vi "test_main.vi"() -> ()   [LabVIEW 2016]
uses:
  AutoBike/Typedef/Remote Control Cluster.ctl
  Downloads/PID Gains.ctl
  LabView Navigation/INS Data.ctl
  <vilib>/FPGAPlugInAG/roboRIO/niLvFpga_Open_roboRIO.vi
  <vilib>/rvi/interface/common/dynamic/niFpgaDynamicAddResources.vi
  <vilib>/FPGAPlugInAG/Dynamic/niLvFpga_Reset_Dynamic.vi
  <vilib>/Utility/error.llb/Error Cluster From Error Code.vi
  <vilib>/rvi/errors/niLvFpgaAdjustHostInterfaceError.vi
  <vilib>/myRIO/Common/Instrument Driver Framework/Utilities/vis/FPGA Ref Manager.vi
  <vilib>/myRIO/Common/Instrument Driver Framework/Utilities/vis/Ref Counter.vi
  <vilib>/FPGAPlugInAG/Dynamic/niLvFpga_Run_Dynamic.vi
  <vilib>/RVI Host/nirviSupport.llb/nirviErrorClusterFromErrorCode.vi
  <vilib>/addons/control/pid/pid.llb/PID (DBL).vi
  <vilib>/Utility/file.llb/Read Delimited Spreadsheet (DBL).vi
  <vilib>/rvi/interface/nirviOpenFPGA/nirviOpenFPGA.xnode
  AutoBike/FPGA Bitfiles/AutoBikeMainFPGAbitfile.lvbitx
  <vilib>/rvi/interface/nirviMethod/nirviMethod.xnode
  <vilib>/rvi/interface/nirviReadWriteControl/nirviReadWriteControl.xnode
  <vilib>/ErrorRing/Error Ring.xnode
  <vilib>/rvi/interface/Simulation/niFpgaSimulationCallBeginRW.vi
  NiFpgaLv.dll
  <vilib>/FPGAPlugInAG/Dynamic/niLvFpga_WriteFifo_Dynamic.vi
  <vilib>/rvi/errors/niLvFpgaMergeErrorWithErrorCode.vi
  <vilib>/rvi/interface/nirviMethod/StockFPGA_InlinedMethodWaitForSingleIRQ.vi
  <vilib>/FPGAPlugInAG/Dynamic/niLvFpga_WaitOnIrq_Dynamic.vi
  <vilib>/FPGAPlugInAG/Dynamic/niLvFpga_AcknowledgeIrq_Dynamic.vi
  <vilib>/addons/control/pid/NI_PID_pid.lvlib
  <vilib>/myRIO/Instrument Drivers/Utilities/Utilities.lvlib
  <vilib>/FPGAPlugInAG/Dynamic/niLvFpga_StartFifo_Dynamic.vi
  <vilib>/FPGAPlugInAG/Dynamic/niLvFpga_ReadFifo_Dynamic.vi
panel:
  out "Increment Lean":i8
  out "PositionData":T1
  out "SteeringAngle(deg)":dbl
  out "all rows":dbl[][](array[numeric])
  out "Delta Heading":dbl
  in  "useUWB":bool=TRUE
  out "X_UWB":dbl
  out "Y_UWB":dbl
  out "Z_UWB":dbl
  in  "Send vel":bool
  out "VEL":u16=850
  in  "resetPID":bool
  in  "PID gains":T2={"proportional gain (Kc)"=-3.418, "integral time (Ti, min)"=45.215, "derivative time (Td, min)"=0.0011} {"derivative time (Td, min)" format="%.8f"; "integral time (Ti, min)" format="%.8f"; "proportional gain (Kc)" format="%.8f"}
  in  "Gear":enum16{"7", "6", "5", "4", "3", "2", "1"}(ring)=enum."4"
  in  "maxDiff":dbl=0.75
  out "km/h":sgl
  out "Setpoint":dbl
  out "Set Roll":dbl(graph)
  out "encoder setpoint":i16(graph)
  out "Roll":sgl(graph)
  in  "Reset Errors":bool
  out "ODrive State":u8
  out "ODrive Errors":u32
  out "ODrive Error Flags":bool[](array[boolean])
  out "Position Axis1":i16
  out "Velocity Axis0":i16
  out "Remote Control Data":T3
  out "Encoder Index Position":i16
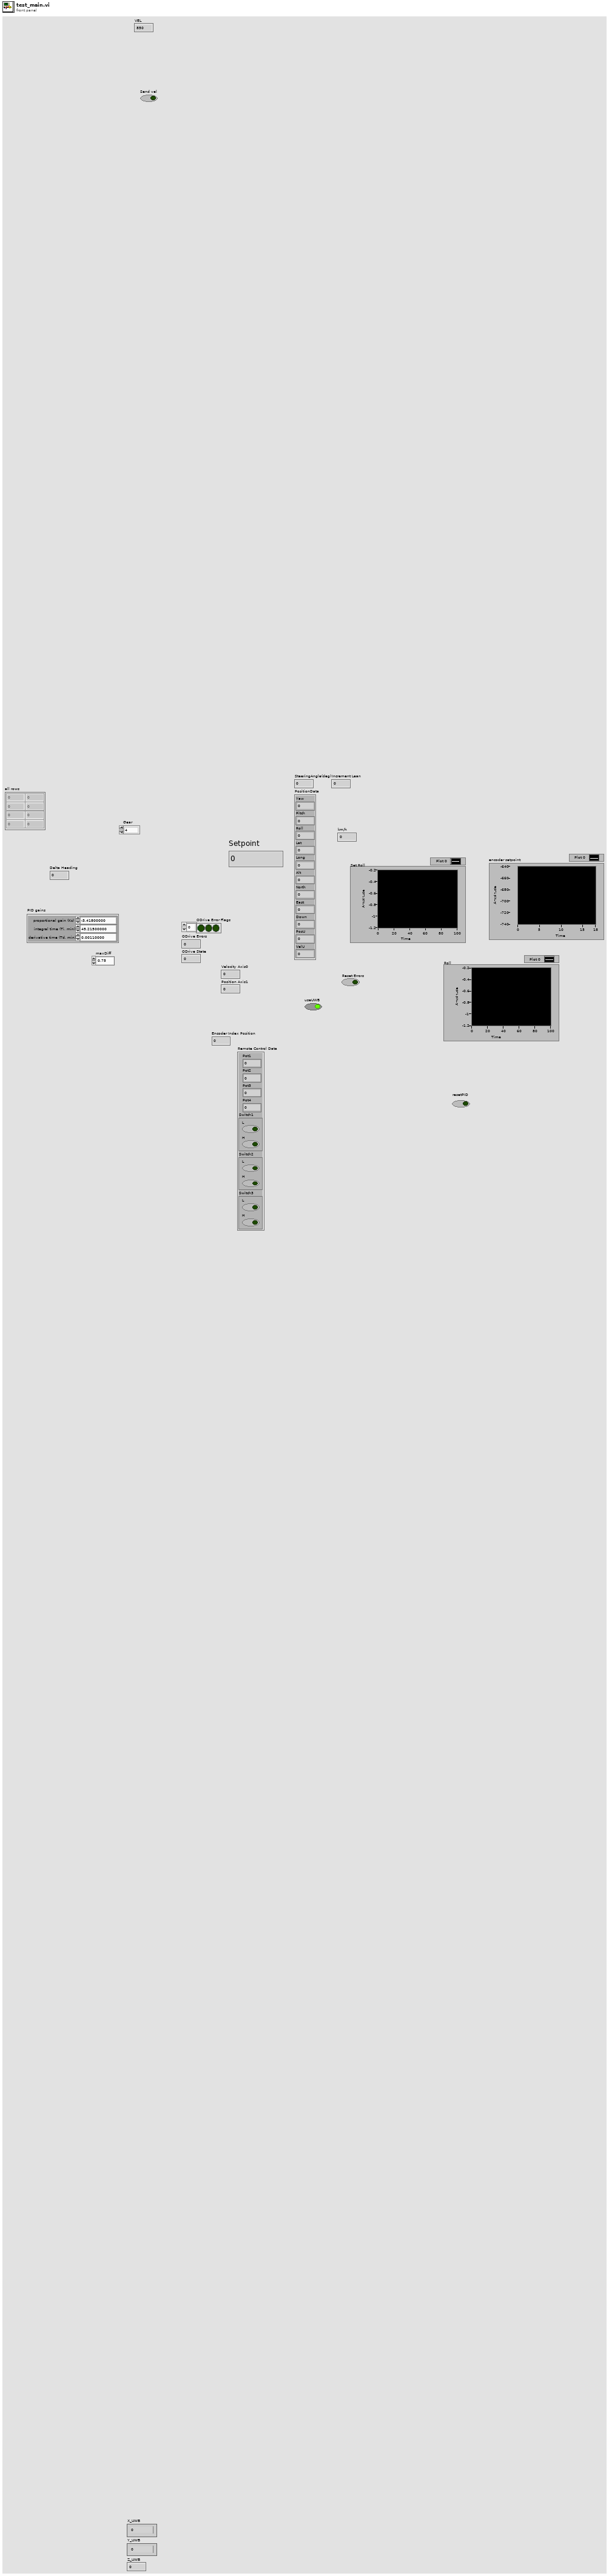
[diagram p1: front panel]
types:
  T1 = typedef "INS Data.ctl" = cluster{"Yaw":sgl, "Pitch":sgl, "Roll":sgl, "Lat":dbl, "Long":dbl, "Alt":dbl, "North":dbl, "East":dbl, "Down":dbl, "PosU":dbl, "VelU":dbl}
  T2 = typedef "PID Gains.ctl" = cluster{"proportional gain (Kc)":dbl, "integral time (Ti, min)":dbl, "derivative time (Td, min)":dbl}
  T3 = typedef "Remote Control Cluster.ctl" = cluster{"Pot1":u16, "Pot2":u16, "Pot3":u16, "Pot4":u16, "Switch1":cluster{"L":bool, "H":bool}, "Switch2":cluster{"L":bool, "H":bool}, "Switch3":cluster{"L":bool, "H":bool}}
  T4 = typedef "Semaphore RefNum" = refnum<k1>
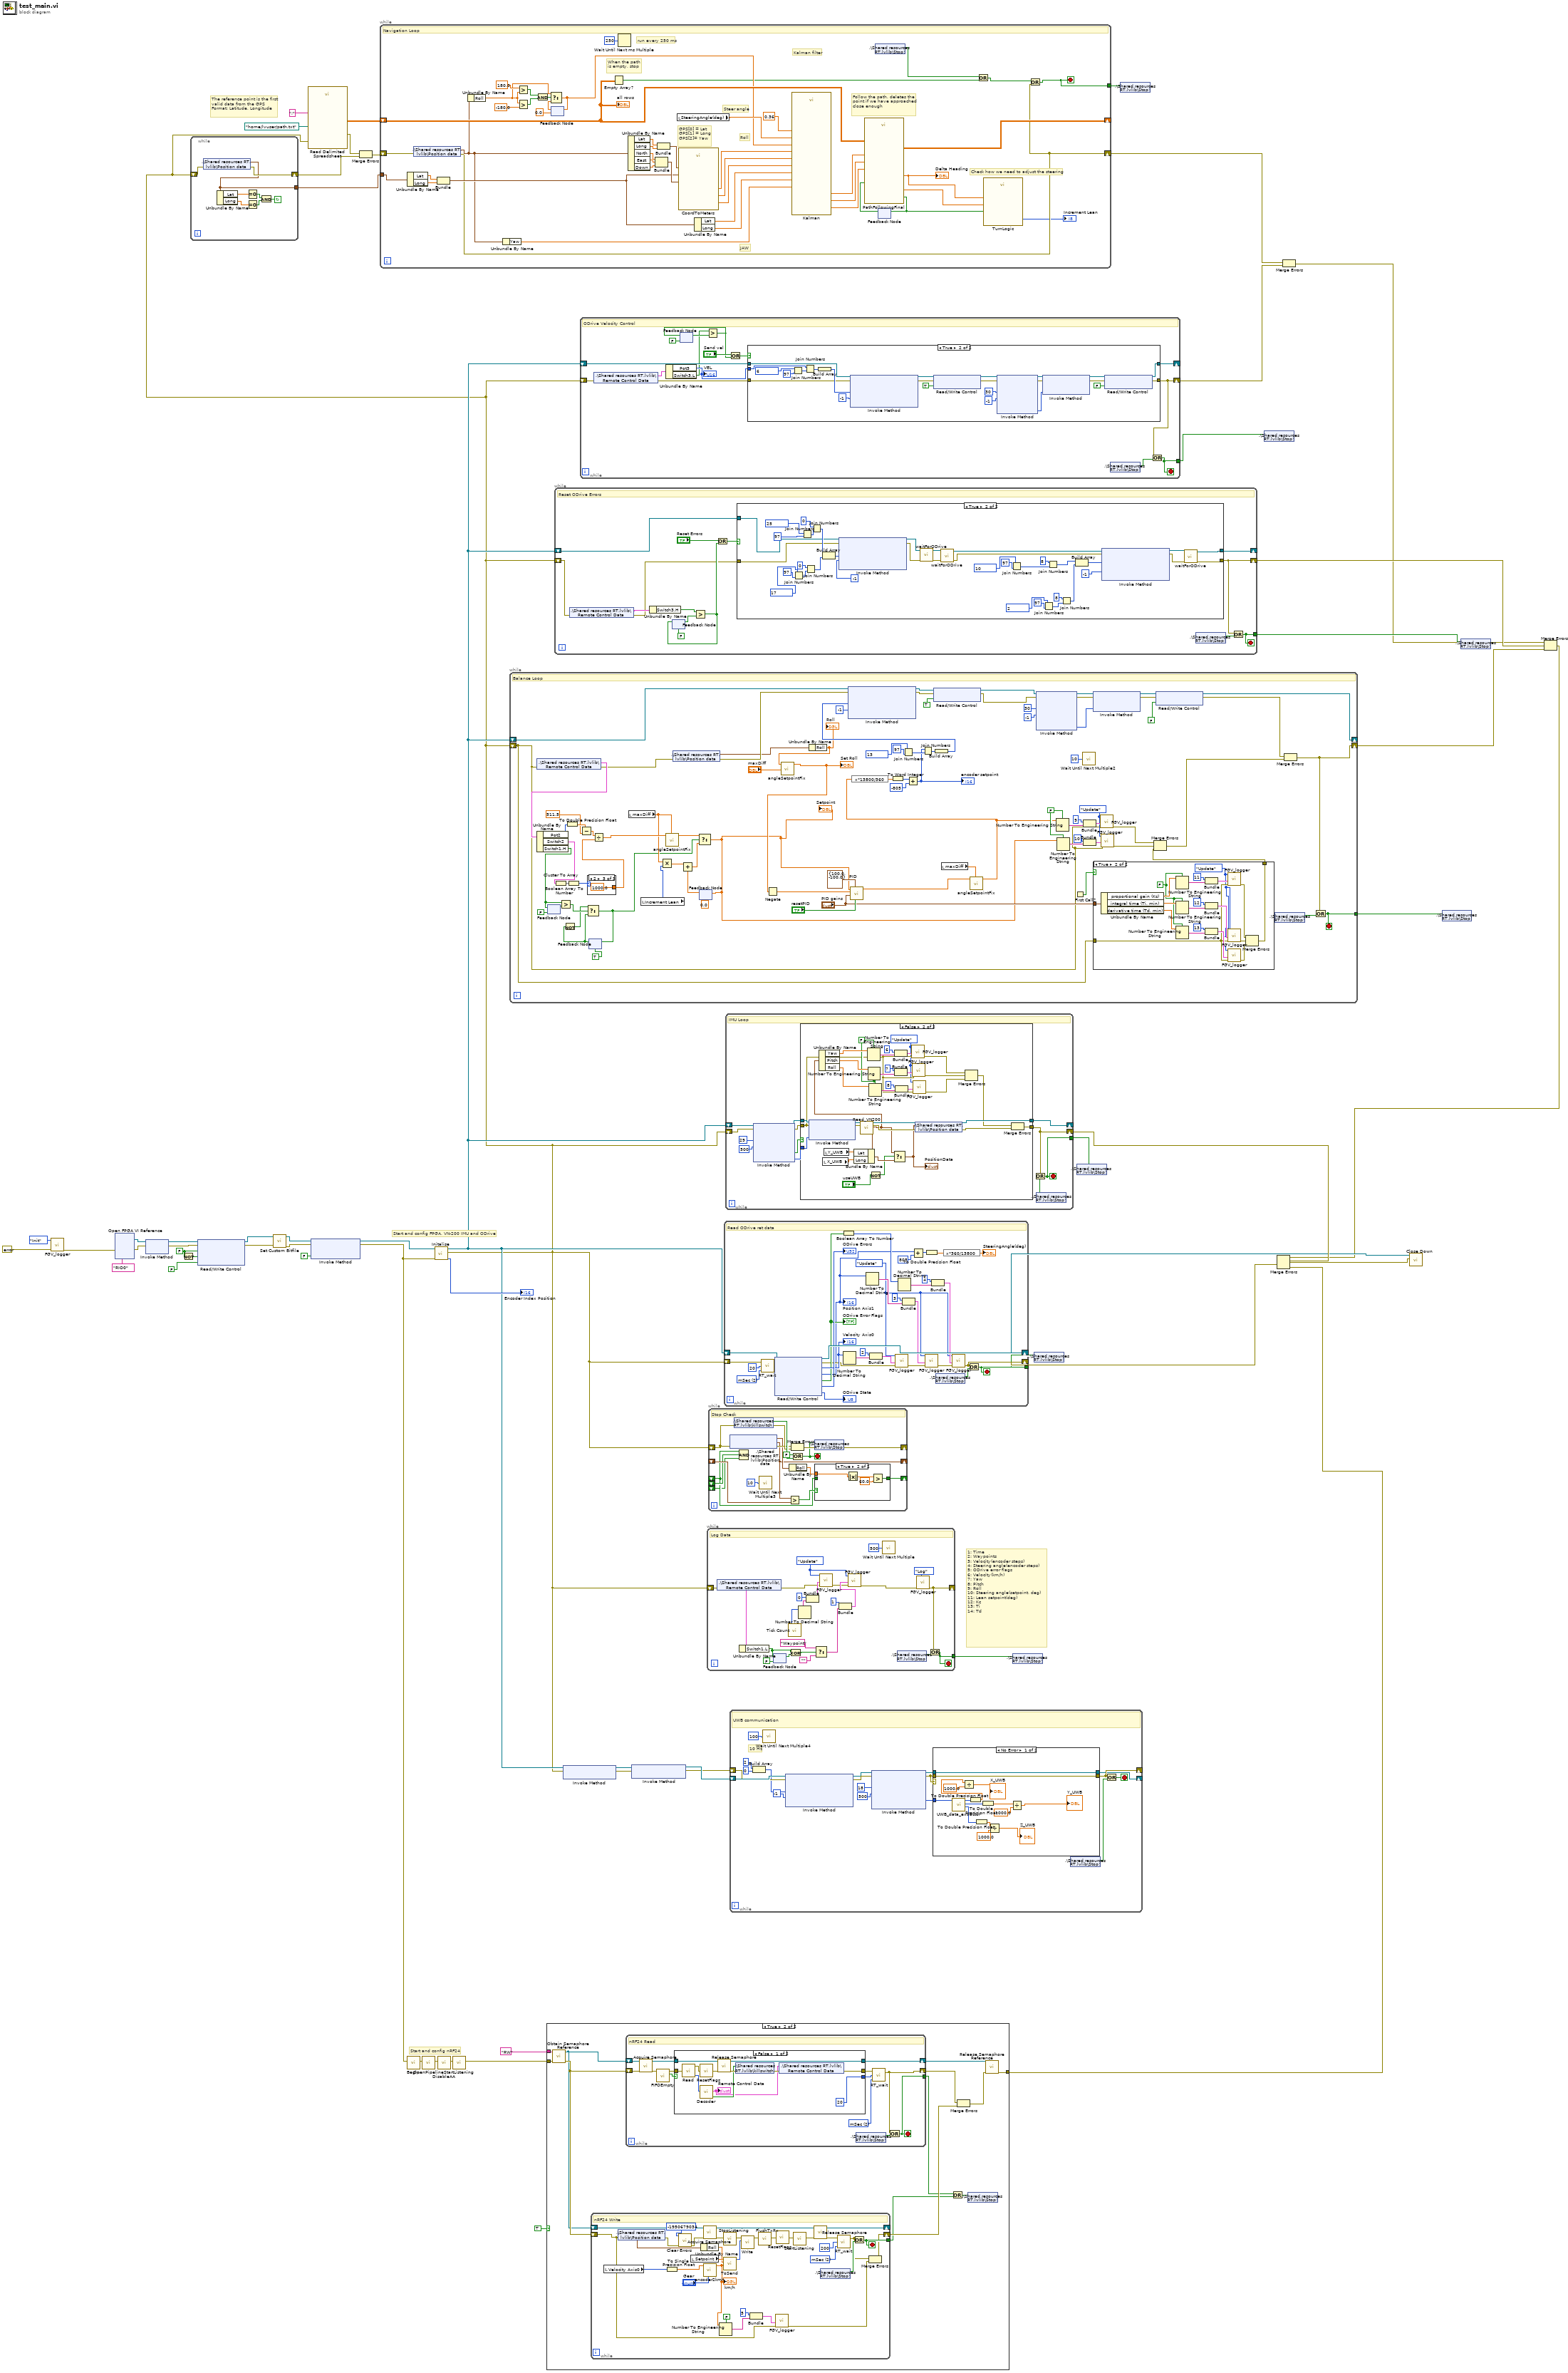
[diagram p0: block diagram]
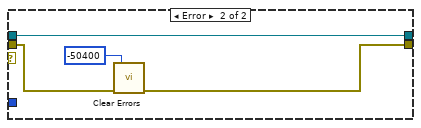
[diagram p2: hidden frame]
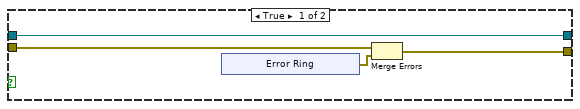
[diagram p3: hidden frame]
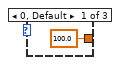
[diagram p8: hidden frame]
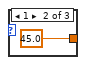
[diagram p9: hidden frame]
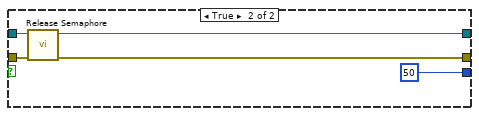
[diagram p11: hidden frame]
diagram:
  w29 = FALSE ("Steering motor on?")
  # "The reference point is the first valid data from the GPS\nFormat: Latitude, Longitude"
  # "1: Time\n2: Waypoints\n3: Velocity(encoder steps)\n4: Steering angle(encoder steps)\n5: ODrive error flags\n6: Velocity(km/h)\n7: Yaw\n8: Pitch\n9: Roll\n10: Steering angle(setpoint, deg)\n11: Lean setpoint(deg)\n12: Kc\n13: Ti\n14: Td"
  # "Start and config FPGA, VN-200 IMU and ODrive"
  # "Start and config nRF24"
  n1 = call "FGV_logger.vi"("error in"=errorcluster {"status"=FALSE, "code"=0, "source"=""}, "Command"=enum16{"Update", "Log", "Init"}."Init") -> ("error out"=w36:errorcluster)  [unwired: 9 in]
  n2 = xnode "Open FPGA VI Reference"("error in"=w36, "resource name"=tag "RIO0") -> ("FPGA VI Reference Out"=w20:refnum<k20>, "error out"=w21:errorcluster)
  n3 = xnode "Invoke Method"("FPGA VI Reference In"=w20, "error in"=w21) -> ("FPGA VI Reference Out"=w33:refnum<k20>, "error out"=w32:errorcluster)
  n4 = Not(x=w29) -> (.not. x?=w30:bool)
  n5 = xnode "Read/Write Control"("FPGA VI Reference In"=w33, "error in"=w32, "Comm LED Green"=w29, "Comm LED Red"=w30, "MotorsON"=FALSE ("Rear wheel motor OFF?")) -> ("FPGA VI Reference Out"=w26:refnum<k20>, "error out"=w27:errorcluster)
  n6 = call <vilib>:"Set Custom Bitfile.vi"("error in (no error)"=w27, "Custom FPGA Reference In"=w26) -> ("error out"=w25:errorcluster, "Custom FPGA Reference Out"=w24:refnum<k20>)  [unwired: 8 in]
  n7 = xnode "Invoke Method"("FPGA VI Reference In"=w24, "error in"=w25, "Wait Until Done (F)"=FALSE) -> ("FPGA VI Reference Out"=w22:refnum<k20>, "error out"=w23:errorcluster)
  n8 = call "Begin.vi"("error in (no error)"=w23) -> ("error out"=w41:errorcluster)  [unwired: 10 in]
  n9 = call "OpenPipeline.vi"("error in (no error)"=w41) -> ("error out"=w40:errorcluster)  [unwired: 10 in]
  n10 = call "Initalise.vi"("error in (no error)"=w23, "FPGA Interface"=w22) -> ("Encoder Index Position"=→"Encoder Index Position":i16, "Error out"=w7:errorcluster, "FPGA VI Reference Out"=w13:refnum<k20>)  [unwired: 7 in]
  n11 = while {
    shift-right: [w64] -> w8
    shift-left: w7 -> [w63]
    tunnel: [w57] -> w9
    stop <- w58 continue-if-true
    n12 = shared-variable ".\\Shared resources RT.lvlib\\Position data"(error in=w63) -> (w57:T1, error out=w64:errorcluster)
    n13 = Unbundle By Name(w57) -> ("Lat"=w62:dbl, "Long"=w61:dbl)
    n14 = Equal To 0?(x=w62) -> (x = 0?=w60:bool)
    n15 = Equal To 0?(x=w61) -> (x = 0?=w59:bool)
    n16 = And(x=w60, y=w59) -> (x .and. y?=w58:bool)
  }
  n17 = call-poly <vilib>:"Read Delimited Spreadsheet.vi"("file path (dialog if empty)"=path "/home/lvuser/path.txt", "error in (no error)"=w7, "delimiter (\\t)"=";" ("delimiter (\\t)")) -> ("all rows"=w10:dbl[][], "error out"=w6:errorcluster)  [unwired: 7 in, 4 out]
  n18 = Merge Errors(w6, w8) -> (w5:errorcluster)
  n19 = while {
    shift-right: [w109] -> _
    shift-left: w10 -> [w97]
    tunnel: w9 -> [w76]
    shift-right: [w70] -> w1
    shift-left: w5 -> [w71]
    tunnel: [w66] -> w4
    stop <- w66 stop-if-true
    # "Roll"
    # "Steer angle"
    # "JAW"
    # "Check how we need to adjust the steering"
    # "Kalman filter"
    # "run every 250 ms"
    # "Follow the path, deletes the point if we have approached close enough"
    # "GPS[0] = Lat\nGPS[1] = Long \nGPS[2]= Yaw"
    # "When the path is empty, stop"
    # "Navigation Loop"
    n20 = Unbundle By Name(w76) -> ("Lat"=w75:dbl, "Long"=w74:dbl)
    n21 = shared-variable ".\\Shared resources RT.lvlib\\Position data"(error in=w71) -> (w72:T1, error out=w70:errorcluster)
    n22 = Bundle("Lat"=w75, "Long"=w74) -> (w73:cluster{"Lat":dbl, "Long":dbl})  [unwired: 1 in]
    n23 = Unbundle By Name(w72) -> ("Roll"=w81:sgl)
    n24 = Unbundle By Name(w72) -> ("Yaw"=w77:sgl)
    n25 = Greater?(x=sgl 180.0 ("upper limit"), y=w81) -> (0:w82:bool)
    n26 = Greater?(x=w81, y=sgl -180.0 ("lower limit")) -> (0:w84:bool)
    n27 = And(x=w82, y=w84) -> (x .and. y?=w83:bool)
    n28 = feedback #1(sgl 0.0 ("Roll")) -> (w80:sgl)
    n29 = Select(t=w81, s=w83, f=w80) -> (s? t:f=w78:sgl)
    n30 = feedback-in #1(w78) -> ()
    n31 = Empty Array?(array=w97) -> (empty?=w69:bool)
    n32 = Wait Until Next ms Multiple(millisecond multiple=u32 250) -> ()  [unwired: 1 out]
    n33 = Unbundle By Name(w72) -> ("Lat"=w104:dbl, "Long"=w103:dbl, "North"=w101:dbl, "East"=w100:dbl, "Down"=w99:dbl)
    n34 = Bundle("North"=w101, "East"=w100, "Down"=w99) -> (w98:cluster{"North":dbl, "East":dbl, "Down":dbl})  [unwired: 1 in]
    n35 = Bundle("Lat"=w104, "Long"=w103) -> (w102:cluster{"Lat":dbl, "Long":dbl})  [unwired: 1 in]
    n36 = local read "SteeringAngle(deg)"() -> (w87:dbl)
    n37 = call "CoordToMeters.vi"("VelNed"=w98, "Ref Point"=w73, "GPS position"=w102) -> ("Bike Heading"=w94:dbl, "X"=w95:dbl, "Y"=w96:dbl)  [unwired: 6 in]
    n38 = Unbundle By Name(w73) -> ("Lat"=w89:dbl, "Long"=w88:dbl)
    n39 = call "Kalman.vi"("x"=w88, "y"=w89, "theta"=w77, "GPS X"=w95, "GPS Y"=w96, "GPS theta"=w94, "ds"=0.36, "phi"=w78, "delta"=w87) -> ("new x"=w91:dbl, "new y"=w92:dbl, "new theta"=w90:dbl)  [unwired: 8 in]
    n40 = shared-variable ".\\Shared resources RT.lvlib\\Stop!"() -> (w67:bool)  [unwired: 1 in, 1 out]
    n41 = feedback #2() -> (w108:bool)  [unwired: 1 in]
    n42 = call "PathFollowingFinal.vi"("GPS_Lat"=w92, "GPS_Long"=w91, "Path"=w97, "Heading angle"=w90, "Save heading"=w108) -> ("Path rest"=w109:dbl[][], "Delta Heading Angle"=w106:dbl, "Goal reached"=w105:bool, "Beta"=w107:dbl)  [unwired: 7 in]
    "Delta Heading" <- w106
    n43 = feedback-in #2(w105) -> ()
    n44 = Or(x=w67, y=w69) -> (x .or. y?=w68:bool)
    n45 = call "TurnLogic.vi"("Goal Reached"=w105, "Beta"=w107, "Delta Theta"=w106) -> ("Increment Lean"=→"Increment Lean":i8)  [unwired: 8 in]
    n46 = Or(x=w68, y=w70) -> (x .or. y?=w66:bool)
    "all rows" <- w97
  }
  n47 = call "DisableAA.vi"("error in (no error)"=w40) -> ("error out"=w39:errorcluster)  [unwired: 10 in]
  n48 = call "StartListening.vi"("error in (no error)"=w39) -> ("error out"=w38:errorcluster)  [unwired: 10 in]
  n49 = while {
    shift-right: [w192] -> _
    shift-left: w13 -> [w193]
    shift-right: [w132] -> w43
    shift-left: w7 -> [w129]
    tunnel: [w154] -> w46
    stop <- w154 stop-if-true
    w138 = enum16{"Update", "Log", "Init"}."Update" ("Command")
    w139 = FALSE ("use system decimal point (T)")
    # "Balance Loop"
    n50 = shared-variable ".\\Shared resources RT.lvlib\\Remote Control Data"(error in=w129) -> (w153:T3, error out=w148:errorcluster)
    n51 = Unbundle By Name(w153) -> ("Pot2"=w189:u16, "Switch2"=w152:cluster{"L":bool, "H":bool}, "Switch1.H"=w118:bool)
    n52 = feedback-in #3(w118) -> ()
    n53 = feedback #3(FALSE ("H")) -> (w117:bool)
    n54 = Cluster To Array(cluster=w152) -> (array=w151:bool[])
    n55 = Greater?(x=w118, y=w117) -> (0:w115:bool)
    n56 = To Double Precision Float(number=w189) -> (double precision float=w187:dbl)
    n57 = Boolean Array To Number(Boolean array=w151) -> (number=w150:u32)
    n58 = Subtract(x=w187, y=511.5 ("x")) -> (x-y=w188:dbl)
    n59 = case shown="2" w150 {
      tunnel: [100.0 45.0 1000.0] -> w149
      frame 0, Default {
      }
      frame 1 {
      }
      frame 2 {
      }
    }
    n60 = feedback #4(TRUE) -> (w113:bool)
    n61 = Not(x=w113) -> (.not. x?=w112:bool)
    n62 = Select(t=w112, s=w115, f=w113) -> (s? t:f=w111:bool)
    n63 = feedback-in #4(w111) -> ()
    n64 = Divide(x=w188, y=w149) -> (x/y=w190:dbl)
    n65 = local read "maxDiff"() -> (w123:dbl)
    n66 = local read "Increment Lean"() -> (w122:i8)
    n67 = Multiply(x=w123, y=w122) -> (x*y=w121:dbl)
    n68 = call "angleSetpointFix.vi"("maxDiff"=w123, "Angle in"=w190) -> ("Angle out"=w126:dbl)  [unwired: 9 in]
    n69 = shared-variable ".\\Shared resources RT.lvlib\\Position data"(error in=w148) -> (w146:T1, error out=w147:errorcluster)
    n70 = feedback #5(0.0 ("Angle out")) -> (w124:dbl)
    n71 = Add(x=w121, y=w124) -> (x+y=w120:dbl)
    n72 = Select(t=w126, s=w111, f=w120) -> (s? t:f=w125:dbl)
    "Setpoint" <- w125
    n73 = feedback-in #5(w125) -> ()
    n74 = Unbundle By Name(w146) -> ("Roll"=w161:sgl)
    "Roll" <- w161
    n75 = call "angleSetpointFix.vi"("maxDiff"="maxDiff", "Angle in"=w161) -> ("Angle out"=w162:dbl)  [unwired: 9 in]
    "Set Roll" <- w162
    n76 = Negate(x=w162) -> (-x=w157:dbl)
    n77 = call-poly <vilib>:"PID.vi"("reinitialize? (F)"="resetPID", "output range"=cluster{"output high":dbl, "output low":dbl} {"output high"=100.0, "output low"=-100.0}, "PID gains"="PID gains", "process variable"=w157, "setpoint"=w125) -> ("output"=w156:dbl)  [unwired: 5 in, 1 out]
    n78 = Join Numbers(hi=u8 13 ("lo"), lo=u8 97) -> ((hi.lo)=w170:u16)
    n79 = local read "maxDiff"() -> (w163:dbl)
    n80 = call "angleSetpointFix.vi"("maxDiff"=w163, "Angle in"=w156) -> ("Angle out"=w135:dbl)  [unwired: 9 in]
    n81 = expression code="x*13800/360"(w135) -> (w164:dbl)
    n82 = To Word Integer(number=w164) -> (16bit integer=w167:i16)
    n83 = Add(x=w167, y=i16 -805 ("hi")) -> (x+y=w165:i16)
    "encoder setpoint" <- w165
    n84 = Join Numbers(hi=w165, lo=w170) -> ((hi.lo)=w169:u32)
    n85 = Build Array(w169) -> (w166:u32[])
    n86 = xnode "Invoke Method"("FPGA VI Reference In"=w193, "error in"=w147, "Data"=w166, "Timeout (ms)"=-1) -> ("FPGA VI Reference Out"=w178:refnum<k20>, "error out"=w179:errorcluster)  [unwired: 1 out]
    n87 = xnode "Read/Write Control"("FPGA VI Reference In"=w178, "error in"=w179, "ODrive RT Control"=TRUE) -> ("FPGA VI Reference Out"=w177:refnum<k20>, "error out"=w176:errorcluster)
    n88 = xnode "Invoke Method"("FPGA VI Reference In"=w177, "error in"=w176, "IRQ Number(s)"=30, "Timeout (ms)"=-1) -> ("FPGA VI Reference Out"=w185:refnum<k20>, "error out"=w184:errorcluster, "IRQ(s) Asserted"=w174:i32)  [unwired: 1 out]
    n89 = Number To Engineering String(1:w139, 4:w135) -> (0:w143:string)  [unwired: 2 in]
    n90 = Number To Engineering String(1:w139, 4:w125) -> (0:w140:string)  [unwired: 2 in]
    n91 = First Call?() -> (First Call?: T/F=w131:bool)
    n92 = call "Wait Until Next Multiple2"("Count(mSec)"=u32 10) -> ()  [unwired: 1 out]
    n93 = Bundle(9, w143) -> (w144:cluster{i32, string})  [unwired: 1 in]
    n94 = Bundle(10, w140) -> (w141:cluster{i32, string})  [unwired: 1 in]
    n95 = case shown="True" w131 {
      tunnel: "PID gains" -> [_ w211]
      tunnel: w129 -> [w194 w200]
      tunnel: [w194 w196] -> w128
      frame False {
      }
      frame True {
        w195 = enum16{"Update", "Log", "Init"}."Update" ("Command")
        w201 = FALSE ("use system decimal point (T)")
        n96 = Unbundle By Name(w211) -> ("proportional gain (Kc)"=w210:dbl, "integral time (Ti, min)"=w203:dbl, "derivative time (Td, min)"=w202:dbl)
        n97 = Number To Engineering String(1:w201, 4:w210) -> (0:w212:string)  [unwired: 2 in]
        n98 = Number To Engineering String(1:w201, 4:w203) -> (0:w207:string)  [unwired: 2 in]
        n99 = Number To Engineering String(1:w201, 4:w202) -> (0:w204:string)  [unwired: 2 in]
        n100 = Bundle(11, w212) -> (w213:cluster{i32, string})  [unwired: 1 in]
        n101 = Bundle(12, w207) -> (w208:cluster{i32, string})  [unwired: 1 in]
        n102 = Bundle(13, w204) -> (w205:cluster{i32, string})  [unwired: 1 in]
        n103 = call "FGV_logger.vi"("error in"=w200, 9:w213, "Command"=w195) -> ("error out"=w199:errorcluster)  [unwired: 8 in]
        n104 = call "FGV_logger.vi"("error in"=w200, 9:w208, "Command"=w195) -> ("error out"=w198:errorcluster)  [unwired: 8 in]
        n105 = call "FGV_logger.vi"("error in"=w200, 9:w205, "Command"=w195) -> ("error out"=w197:errorcluster)  [unwired: 8 in]
        n106 = Merge Errors(w199, w198, w197) -> (w196:errorcluster)
      }
    }
    n107 = xnode "Invoke Method"("FPGA VI Reference In"=w185, "error in"=w184, "IRQ Number(s)"=w174) -> ("FPGA VI Reference Out"=w182:refnum<k20>, "error out"=w173:errorcluster)
    n108 = call "FGV_logger.vi"("error in"=w129, 9:w144, "Command"=w138) -> ("error out"=w137:errorcluster)  [unwired: 8 in]
    n109 = call "FGV_logger.vi"("error in"=w129, 9:w141, "Command"=w138) -> ("error out"=w136:errorcluster)  [unwired: 8 in]
    n110 = Merge Errors(w137, w136, w128) -> (w133:errorcluster)
    n111 = xnode "Read/Write Control"("FPGA VI Reference In"=w182, "error in"=w173, "ODrive RT Control"=FALSE) -> ("FPGA VI Reference Out"=w192:refnum<k20>, "error out"=w134:errorcluster)
    n112 = shared-variable ".\\Shared resources RT.lvlib\\Stop!"() -> (w155:bool)  [unwired: 1 in, 1 out]
    n113 = Merge Errors(w134, w133) -> (w132:errorcluster)
    n114 = Or(x=w132, y=w155) -> (x .or. y?=w154:bool)
  }
  n115 = case shown="True" TRUE {
    tunnel: "RW" ("name (unnamed)") -> [_ w230]
    tunnel: w38 -> [w218 w227]
    tunnel: [w218 w226] -> w51
    frame False {
    }
    frame True {
      n116 = call <vilib>:"Obtain Semaphore Reference.vi"("error in (no error)"=w227, "name (unnamed)"=w230) -> ("error out"=w229:errorcluster, "semaphore"=w228:T4)  [unwired: 3 in, 1 out]
      n117 = while {
        shift-right: [w257] -> _
        shift-left: w228 -> [w263]
        shift-right: [w235] -> w224
        shift-left: w229 -> [w237]
        tunnel: [w244] -> w220
        stop <- w244 stop-if-true
        w254 = u16 2 items=["Ticks", "uSec", "mSec"] ("Counter Units")
        # "nRF24 Write"
        n118 = local read "Velocity Axis0"() -> (w251:i16)
        n119 = shared-variable ".\\Shared resources RT.lvlib\\Position data"(error in=w237) -> (w243:T1, error out=w233:errorcluster)
        n120 = To Single Precision Float(number=w251) -> (single precision float=w250:sgl)
        n121 = call <vilib>:"Clear Errors.vi"("error in (no error)"=w233, "specific error code to clear (0: all)"=-1950679034) -> ("error out"=w232:errorcluster)  [unwired: 4 in, 1 out]
        n122 = local read "Setpoint"() -> (w253:dbl)
        n123 = Unbundle By Name(w243) -> ("Roll"=w252:sgl)
        n124 = call <vilib>:"Acquire Semaphore.vi"("error in (no error)"=w232, "semaphore"=w263) -> ("error out"=w262:errorcluster, "semaphore out"=w258:T4)  [unwired: 3 in, 1 out]
        n125 = call "encoder2kmh.vi"("Gear"="Gear", "encoderSpeed"=w250) -> ("realVelocity"=w240:sgl)  [unwired: 9 in]
        "km/h" <- w240
        n126 = Number To Engineering String(1:FALSE ("use system decimal point (T)"), 4:w240) -> (0:w238:string)  [unwired: 2 in]
        n127 = call "StopListening.vi"("error in (no error)"=w262) -> ("error out"=w248:errorcluster)  [unwired: 10 in]
        n128 = call "ToSend.vi"("velocity"=w240, "leanAngel"=w252, "setpoint"=w253) -> ("data2nRF24"=w246:u8[])  [unwired: 8 in]
        n129 = call "Write.vi"("Input"=w246, "error in (no error)"=w248) -> ("error out"=w247:errorcluster)  [unwired: 8 in, 1 out]
        n130 = Bundle(5, w238) -> (w241:cluster{i32, string})  [unwired: 1 in]
        n131 = call "FlushTxRx.vi"("error in (no error)"=w247) -> ("error out"=w261:errorcluster)  [unwired: 10 in]
        n132 = call "FGV_logger.vi"("error in"=w237, 9:w241) -> ("error out"=w234:errorcluster)  [unwired: 9 in]
        n133 = call "ResetFlags.vi"("error in (no error)"=w261) -> ("error out"=w260:errorcluster)
        n134 = call "StartListening.vi"("error in (no error)"=w260) -> ("error out"=w259:errorcluster)  [unwired: 10 in]
        n135 = call <vilib>:"Release Semaphore.vi"("error in (no error)"=w259, "semaphore"=w258) -> ("error out"=w256:errorcluster, "semaphore out"=w257:T4)  [unwired: 4 in]
        n136 = shared-variable ".\\Shared resources RT.lvlib\\Stop!"() -> (w245:bool)  [unwired: 1 in, 1 out]
        n137 = call "RT_wait.vi"("Counter Units"=w254, "Count(mSec)"=u32 200 ("Count(uSec)"), "error in (no error)"=w256) -> ("error out"=w236:errorcluster)  [unwired: 1 in, 1 out]
        n138 = Or(x=w236, y=w245) -> (x .or. y?=w244:bool)
        n139 = Merge Errors(w236, w234) -> (w235:errorcluster)
      }
      n140 = while {
        shift-right: [w271] -> w225
        shift-left: w228 -> [w276]
        shift-right: [w265] -> w223
        shift-left: w229 -> [w275]
        tunnel: [w264] -> w219
        stop <- w264 stop-if-true
        w268 = u16 2 items=["Ticks", "uSec", "mSec"] ("Counter Units")
        # "nRF24 Read"
        n141 = call <vilib>:"Acquire Semaphore.vi"("error in (no error)"=w275, "semaphore"=w276) -> ("error out"=w274:errorcluster, "semaphore out"=w272:T4)  [unwired: 3 in, 1 out]
        n142 = call "FIFOEmpty.vi"("error in (no error)"=w274) -> ("RX_EMPTY"=w270:bool, "error out"=w273:errorcluster)  [unwired: 9 in]
        n143 = case shown="False" w270 {
          tunnel: w273 -> [w288 w293]
          tunnel: w272 -> [w285 w292]
          tunnel: [w277 w290] -> w269
          tunnel: [w284 w291] -> w271
          tunnel: [u32 20 ("Count(uSec)") u32 50 ("Count(uSec)")] -> w267
          frame False {
            n144 = call "Read.vi"("error in (no error)"=w288) -> ("error out"=w287:errorcluster, "Data frame"=w283:u16[])  [unwired: 1 out]
            n145 = call "ResetFlags.vi"("error in (no error)"=w287) -> ("error out"=w286:errorcluster)
            n146 = call "Decoder.vi"("Data frame"=w283) -> ("output cluster"=w278:T3, "Kill Switch"=w280:bool)  [unwired: 17 in]
            "Remote Control Data" <- w278
            n147 = call <vilib>:"Release Semaphore.vi"("error in (no error)"=w286, "semaphore"=w285) -> ("error out"=w281:errorcluster, "semaphore out"=w284:T4)  [unwired: 4 in]
            n148 = shared-variable ".\\Shared resources RT.lvlib\\killswitch"(w280, error in=w281) -> (error out=w279:errorcluster)
            n149 = shared-variable ".\\Shared resources RT.lvlib\\Remote Control Data"(w278, error in=w279) -> (error out=w277:errorcluster)
          }
          frame True {
            n150 = call <vilib>:"Release Semaphore.vi"("error in (no error)"=w293, "semaphore"=w292) -> ("error out"=w290:errorcluster, "semaphore out"=w291:T4)  [unwired: 4 in]
          }
        }
        n151 = shared-variable ".\\Shared resources RT.lvlib\\Stop!"() -> (w266:bool)  [unwired: 1 in, 1 out]
        n152 = call "RT_wait.vi"("Counter Units"=w268, "Count(mSec)"=w267, "error in (no error)"=w269) -> ("error out"=w265:errorcluster)  [unwired: 1 in, 1 out]
        n153 = Or(x=w265, y=w266) -> (x .or. y?=w264:bool)
      }
      n154 = Or(x=w219, y=w220) -> (x .or. y?=w221:bool)
      n155 = Merge Errors(w223, w224) -> (w222:errorcluster)
      n156 = shared-variable ".\\Shared resources RT.lvlib\\Stop!"(w221) -> ()  [unwired: 1 in, 1 out]
      n157 = call <vilib>:"Release Semaphore Reference.vi"("error in (no error)"=w222, "semaphore"=w225) -> ("error out"=w226:errorcluster)  [unwired: 8 in, 1 out]
    }
  }
  n158 = while {
    shift-right: [w306] -> _
    shift-left: w13 -> [w307]
    shift-right: [w295] -> w44
    shift-left: w7 -> [w297]
    tunnel: [w294] -> w47
    stop <- w294 stop-if-true
    # "Reset ODrive Errors"
    n159 = shared-variable ".\\Shared resources RT.lvlib\\Remote Control Data"(error in=w297) -> (w299:T3, error out=w298:errorcluster)
    n160 = Unbundle By Name(w299) -> ("Switch3.H"=w305:bool)
    n161 = feedback #6(FALSE) -> (w304:bool)
    n162 = Greater?(x=w305, y=w304) -> (0:w302:bool)
    n163 = feedback-in #6(w302) -> ()
    n164 = Or(x="Reset Errors", y=w302) -> (x .or. y?=w300:bool)
    n165 = case shown="True" w300 {
      tunnel: w307 -> [w309 w329]
      tunnel: w298 -> [w308 w328]
      tunnel: [w309 w311] -> w306
      tunnel: [w308 w310] -> w295
      frame False {
      }
      frame True {
        n166 = Join Numbers(hi=u8 17 ("lo"), lo=u8 97) -> ((hi.lo)=w334:u16)
        n167 = Join Numbers(hi=u8 25 ("lo"), lo=u8 97) -> ((hi.lo)=w345:u16)
        n168 = Join Numbers(hi=u16 0, lo=w334) -> ((hi.lo)=w332:u32)
        n169 = Join Numbers(hi=u16 0, lo=w345) -> ((hi.lo)=w343:u32)
        n170 = Build Array(w343, w332) -> (w342:u32[])
        n171 = xnode "Invoke Method"("FPGA VI Reference In"=w329, "error in"=w328, "Data"=w342, "Timeout (ms)"=-1) -> ("FPGA VI Reference Out"=w339:refnum<k20>, "error out"=w340:errorcluster)  [unwired: 1 out]
        n172 = call "waitForODrive.vi"("error in (no error)"=w340, "Refnum in"=w339) -> ("error out"=w331:errorcluster, "Refnum out"=w330:refnum<k20>)  [unwired: 8 in]
        n173 = call "waitForODrive.vi"("error in (no error)"=w331, "Refnum in"=w330) -> ("error out"=w314:errorcluster, "Refnum out"=w315:refnum<k20>)  [unwired: 8 in]
        n174 = Join Numbers(hi=u8 10 ("lo"), lo=u8 97) -> ((hi.lo)=w324:u16)
        n175 = Join Numbers(hi=u8 2 ("lo"), lo=u8 97) -> ((hi.lo)=w320:u16)
        n176 = Join Numbers(hi=u16 8, lo=w324) -> ((hi.lo)=w326:u32)
        n177 = Join Numbers(hi=u16 8, lo=w320) -> ((hi.lo)=w317:u32)
        n178 = Build Array(w326, w317) -> (w327:u32[])
        n179 = xnode "Invoke Method"("FPGA VI Reference In"=w315, "error in"=w314, "Data"=w327, "Timeout (ms)"=-1) -> ("FPGA VI Reference Out"=w313:refnum<k20>, "error out"=w312:errorcluster)  [unwired: 1 out]
        n180 = call "waitForODrive.vi"("error in (no error)"=w312, "Refnum in"=w313) -> ("error out"=w310:errorcluster, "Refnum out"=w311:refnum<k20>)  [unwired: 8 in]
      }
    }
    n181 = shared-variable ".\\Shared resources RT.lvlib\\Stop!"() -> (w296:bool)  [unwired: 1 in, 1 out]
    n182 = Or(x=w295, y=w296) -> (x .or. y?=w294:bool)
  }
  n183 = xnode "Invoke Method"("FPGA VI Reference In"=w13, "error in"=w7) -> ("FPGA VI Reference Out"=w17:refnum<k20>, "error out"=w16:errorcluster)
  n184 = while {
    shift-right: [w360] -> _
    shift-left: w13 -> [w359]
    shift-right: [w347] -> w3
    shift-left: w7 -> [w351]
    tunnel: [w346] -> w18
    stop <- w346 stop-if-true
    # "ODrive Velocity Control"
    n185 = shared-variable ".\\Shared resources RT.lvlib\\Remote Control Data"(error in=w351) -> (w349:T3, error out=w350:errorcluster)
    n186 = Unbundle By Name(w349) -> ("Pot3"=w358:u16, "Switch3.L"=w352:bool)
    "VEL" <- w358
    n187 = feedback #7(FALSE) -> (w355:bool)
    n188 = Greater?(x=w352, y=w355) -> (0:w356:bool)
    n189 = feedback-in #7(w356) -> ()
    n190 = Or(x="Send vel", y=w356) -> (x .or. y?=w353:bool)
    n191 = case shown="True" w353 {
      tunnel: w358 -> [_ w367]
      tunnel: [w362 w366] -> w347
      tunnel: [w361 w365] -> w360
      tunnel: w350 -> [w362 w364]
      tunnel: w359 -> [w361 w363]
      frame False {
      }
      frame True {
        n192 = Join Numbers(hi=u8 6 ("lo"), lo=u8 97) -> ((hi.lo)=w371:u16)
        n193 = Join Numbers(hi=w367, lo=w371) -> ((hi.lo)=w370:u32)
        n194 = Build Array(w370) -> (w368:u32[])
        n195 = xnode "Invoke Method"("FPGA VI Reference In"=w363, "error in"=w364, "Data"=w368, "Timeout (ms)"=-1) -> ("FPGA VI Reference Out"=w375:refnum<k20>, "error out"=w376:errorcluster)  [unwired: 1 out]
        n196 = xnode "Read/Write Control"("FPGA VI Reference In"=w375, "error in"=w376, "ODrive RT Control"=TRUE) -> ("FPGA VI Reference Out"=w374:refnum<k20>, "error out"=w373:errorcluster)
        n197 = xnode "Invoke Method"("FPGA VI Reference In"=w374, "error in"=w373, "IRQ Number(s)"=30, "Timeout (ms)"=-1) -> ("FPGA VI Reference Out"=w385:refnum<k20>, "error out"=w382:errorcluster, "IRQ(s) Asserted"=w383:i32)  [unwired: 1 out]
        n198 = xnode "Invoke Method"("FPGA VI Reference In"=w385, "error in"=w382, "IRQ Number(s)"=w383) -> ("FPGA VI Reference Out"=w380:refnum<k20>, "error out"=w379:errorcluster)
        n199 = xnode "Read/Write Control"("FPGA VI Reference In"=w380, "error in"=w379, "ODrive RT Control"=FALSE) -> ("FPGA VI Reference Out"=w365:refnum<k20>, "error out"=w366:errorcluster)
      }
    }
    n200 = shared-variable ".\\Shared resources RT.lvlib\\Stop!"() -> (w348:bool)  [unwired: 1 in, 1 out]
    n201 = Or(x=w347, y=w348) -> (x .or. y?=w346:bool)
  }
  n202 = xnode "Invoke Method"("FPGA VI Reference In"=w17, "error in"=w16) -> ("FPGA VI Reference Out"=w15:refnum<k20>, "error out"=w14:errorcluster)
  n203 = while {
    tunnel: [w409] -> w34
    shift-right: [w403] -> _
    shift-left: w7 -> [w400]
    stop <- w409 stop-if-true
    w402 = enum16{"Update", "Log", "Init"}."Update" ("Command")
    # "Log Data"
    n204 = shared-variable ".\\Shared resources RT.lvlib\\Remote Control Data"(error in=w400) -> (w398:T3, error out=w399:errorcluster)
    n205 = Unbundle By Name(w398) -> ("Switch1.L"=w387:bool)
    n206 = feedback-in #8(w387) -> ()
    n207 = feedback #8(FALSE ("L")) -> (w389:bool)
    n208 = call "Tick Count"() -> ("Tick Count(mSec)"=w404:u32)
    n209 = Exclusive Or(1:w389, 2:w387) -> (0:w388:bool)
    n210 = Number To Decimal String(number=w404) -> (decimal integer string=w405:string)  [unwired: 1 in]
    n211 = Bundle(0, w405) -> (w407:cluster{i32, string})  [unwired: 1 in]
    n212 = Select(t="Waypoint", s=w388, f="") -> (s? t:f=w394:string)
    n213 = call "FGV_logger.vi"("error in"=w399, 9:w407, "Command"=w402) -> ("error out"=w392:errorcluster)  [unwired: 8 in]
    n214 = Bundle(1, "t"=w394) -> (w393:cluster{i32, "t":string})  [unwired: 1 in]
    n215 = call "FGV_logger.vi"("error in"=w392, 9:w393, "Command"=w402) -> ("error out"=w391:errorcluster)  [unwired: 8 in]
    n216 = call "Wait Until Next Multiple"("Count(mSec)"=u32 500) -> ()  [unwired: 1 out]
    n217 = shared-variable ".\\Shared resources RT.lvlib\\Stop!"() -> (w410:bool)  [unwired: 1 in, 1 out]
    n218 = call "FGV_logger.vi"("error in"=w391, "Command"=enum16{"Update", "Log", "Init"}."Log") -> ("error out"=w403:errorcluster)  [unwired: 9 in]
    n219 = Or(x=w403, y=w410) -> (x .or. y?=w409:bool)
  }
  n220 = while {
    shift-right: [w428] -> _
    shift-left: w7 -> [w424]
    shift-right: [w419] -> _
    shift-left: _ -> [w418]
    shift-right: [w415] -> _
    shift-left: _ -> [w413]
    shift-left: _ -> [w414]
    shift-left: _ -> [w412]
    stop <- w421 stop-if-true
    # "Stop Check"
    n221 = shared-variable ".\\Shared resources RT.lvlib\\Position data"(error in=w424) -> (w422:T1, error out=w423:errorcluster, w419:timestamp)
    n222 = shared-variable ".\\Shared resources RT.lvlib\\killswitch"(error in=w424) -> (w427:bool, error out=w425:errorcluster)
    n223 = Compound Arithmetic op=AND(w413, w414, w412) -> ()  [unwired: 1 out]
    n224 = call "Wait Until Next Multiple3"("Count(mSec)"=u32 10) -> ()  [unwired: 1 out]
    n225 = Greater?(x=w419, y=w418) -> (0:w417:bool)
    n226 = Unbundle By Name(w422) -> ("Roll"=w416:sgl)
    n227 = Merge Errors(w423, w425) -> (w426:errorcluster)
    n228 = Compound Arithmetic op=OR(FALSE ("value"), w427) -> (w421:bool)
    n229 = shared-variable ".\\Shared resources RT.lvlib\\Stop!"(w421, error in=w426) -> (error out=w428:errorcluster)
    n230 = case shown="True" w417 {
      tunnel: w416 -> [_ w431]
      tunnel: [w429 w430] -> w415
      tunnel: w413 -> [w429 _]
      frame False {
      }
      frame True {
        n231 = Absolute Value(x=w431) -> (abs(x)=w433:sgl)
        n232 = Greater?(x=w433, y=sgl 60.0) -> (0:w430:bool)
      }
    }
  }
  n233 = while {
    shift-right: [w465] -> w49
    shift-left: w13 -> [w464]
    shift-right: [w439] -> w52
    shift-left: w7 -> [w463]
    tunnel: [w456] -> w45
    stop <- w456 stop-if-true
    w441 = enum16{"Update", "Log", "Init"}."Update" ("Command")
    w460 = u16 2 items=["Ticks", "uSec", "mSec"] ("Counter Units")
    # "Read ODrive ret data"
    n234 = call "RT_wait.vi"("Counter Units"=w460, "Count(mSec)"=u32 20, "error in (no error)"=w463) -> ("error out"=w462:errorcluster)  [unwired: 1 in, 1 out]
    n235 = xnode "Read/Write Control"("FPGA VI Reference In"=w464, "error in"=w462) -> ("FPGA VI Reference Out"=w465:refnum<k20>, "error out"=w440:errorcluster, "Velocity Axis0"=w452:i16, "Position Axis1"=w437:i16, "ODrive Error Flags"=w443:bool[], "ODrive Errors"=→"ODrive Errors":u32, "ODrive State"=→"ODrive State":u8)
    "Velocity Axis0" <- w452
    "Position Axis1" <- w437
    "ODrive Error Flags" <- w443
    n236 = Boolean Array To Number(Boolean array=w443) -> (number=w444:u8)
    n237 = Number To Decimal String(number=w452) -> (decimal integer string=w454:string)  [unwired: 1 in]
    n238 = Number To Decimal String(number=w437) -> (decimal integer string=w450:string)  [unwired: 1 in]
    n239 = Bundle(2, w454) -> (w453:cluster{i32, string})  [unwired: 1 in]
    n240 = call "FGV_logger.vi"("error in"=w440, 9:w453, "Command"=w441) -> ("error out"=w448:errorcluster)  [unwired: 8 in]
    n241 = Number To Decimal String(number=w444) -> (decimal integer string=w446:string)  [unwired: 1 in]
    n242 = Bundle(3, w450) -> (w449:cluster{i32, string})  [unwired: 1 in]
    n243 = Add(x=w437, y=i16 805 ("hi")) -> (x+y=w436:i16)
    n244 = call "FGV_logger.vi"("error in"=w448, 9:w449, "Command"=w441) -> ("error out"=w442:errorcluster)  [unwired: 8 in]
    n245 = To Double Precision Float(number=w436) -> (double precision float=w435:dbl)
    n246 = Bundle(4, w446) -> (w445:cluster{i32, string})  [unwired: 1 in]
    n247 = shared-variable ".\\Shared resources RT.lvlib\\Stop!"() -> (w457:bool)  [unwired: 1 in, 1 out]
    n248 = expression code="x*360/13800"(w435) -> (→"SteeringAngle(deg)":dbl)
    n249 = call "FGV_logger.vi"("error in"=w442, 9:w445, "Command"=w441) -> ("error out"=w439:errorcluster)  [unwired: 8 in]
    n250 = Or(x=w439, y=w457) -> (x .or. y?=w456:bool)
  }
  n251 = while {
    shift-right: [w475] -> w53
    shift-left: w7 -> [w473]
    shift-right: [w477] -> _
    shift-left: w13 -> [w472]
    tunnel: [w474] -> w19
    stop <- w474 stop-if-true
    # "IMU Loop"
    n252 = xnode "Invoke Method"("FPGA VI Reference In"=w472, "error in"=w473, "IRQ Number(s)"=29, "Timeout (ms)"=500) -> ("FPGA VI Reference Out"=w467:refnum<k20>, "error out"=w468:errorcluster, "Timed Out"=w469:bool, "IRQ(s) Asserted"=w466:i32)
    n253 = case shown="False" w469 {
      tunnel: w468 -> [w480 w500]
      tunnel: w467 -> [w481 w518]
      tunnel: [w481 w520] -> w477
      tunnel: [w479 w514] -> w475
      tunnel: w466 -> [_ w516]
      frame True {
        n254 = xnode "Error Ring"() -> ("error out"=w478:errorcluster)
        n255 = Merge Errors(w480, w478) -> (w479:errorcluster)
      }
      frame False {
        w499 = enum16{"Update", "Log", "Init"}."Update" ("Command")
        w503 = FALSE ("use system decimal point (T)")
        n256 = xnode "Invoke Method"("FPGA VI Reference In"=w518, "error in"=w500, "IRQ Number(s)"=w516) -> ("FPGA VI Reference Out"=w488:refnum<k20>, "error out"=w517:errorcluster)
        n257 = local read "X_UWB"() -> (w493:dbl)
        n258 = local read "Y_UWB"() -> (w494:dbl)
        n259 = call "Read_VN200.vi"("FPGA Interface"=w488, "error in"=w517) -> ("FPGA Interface Out"=w520:refnum<k20>, "error out"=w519:errorcluster, "Position Data"=w491:T1)  [unwired: 11 in]
        n260 = Unbundle By Name(w491) -> ("Yaw"=w510:sgl, "Pitch"=w506:sgl, "Roll"=w502:sgl)
        n261 = Bundle By Name(cluster=w491, "Lat"=w494, "Long"=w493) -> (w492:T1)
        n262 = Number To Engineering String(1:w503, 4:w510) -> (0:w511:string)  [unwired: 2 in]
        n263 = Number To Engineering String(1:w503, 4:w506) -> (0:w507:string)  [unwired: 2 in]
        n264 = Number To Engineering String(1:w503, 4:w502) -> (0:w504:string)  [unwired: 2 in]
        n265 = Not(x="useUWB") -> (.not. x?=w489:bool)
        n266 = Select(t=w491, s=w489, f=w492) -> (s? t:f=w487:T1)
        "PositionData" <- w487
        n267 = Bundle(6, w511) -> (w512:cluster{i32, string})  [unwired: 1 in]
        n268 = Bundle(7, w507) -> (w508:cluster{i32, string})  [unwired: 1 in]
        n269 = Bundle(8, w504) -> (w505:cluster{i32, string})  [unwired: 1 in]
        n270 = call "FGV_logger.vi"("error in"=w500, 9:w512, "Command"=w499) -> ("error out"=w498:errorcluster)  [unwired: 8 in]
        n271 = call "FGV_logger.vi"("error in"=w500, 9:w508, "Command"=w499) -> ("error out"=w497:errorcluster)  [unwired: 8 in]
        n272 = call "FGV_logger.vi"("error in"=w500, 9:w505, "Command"=w499) -> ("error out"=w496:errorcluster)  [unwired: 8 in]
        n273 = shared-variable ".\\Shared resources RT.lvlib\\Position data"(w487, error in=w519) -> (error out=w515:errorcluster)
        n274 = Merge Errors(w498, w497, w496) -> (w495:errorcluster)
        n275 = Merge Errors(w495, w515) -> (w514:errorcluster)
      }
    }
    n276 = shared-variable ".\\Shared resources RT.lvlib\\Stop!"() -> (w476:bool)  [unwired: 1 in, 1 out]
    n277 = Or(x=w475, y=w476) -> (x .or. y?=w474:bool)
  }
  n278 = while {
    shift-right: [w521] -> _
    shift-left: w15 -> [w537]
    shift-right: [w525] -> _
    shift-left: w14 -> [w531]
    stop <- w532 stop-if-true
    # "10 Hz"
    # "UWB communication"
    n279 = Build Array(u8 2, u8 0) -> (w527:u8[])
    n280 = call "Wait Until Next Multiple4"("Count(mSec)"=u32 100) -> ()  [unwired: 1 out]
    n281 = xnode "Invoke Method"("FPGA VI Reference In"=w537, "error in"=w531, "Data"=w527, "Timeout (ms)"=-1) -> ("FPGA VI Reference Out"=w534:refnum<k20>, "error out"=w535:errorcluster)  [unwired: 1 out]
    n282 = xnode "Invoke Method"("FPGA VI Reference In"=w534, "error in"=w535, "Number of Elements"=u32 18, "Timeout (ms)"=500) -> ("FPGA VI Reference Out"=w522:refnum<k20>, "error out"=w524:errorcluster, "Data"=w523:u8[])  [unwired: 1 out]
    n283 = case shown="No Error" w524 {
      tunnel: w523 -> [w553 _]
      tunnel: w524 -> [w552 w557]
      tunnel: [w552 w556] -> w525
      tunnel: [w551 w554] -> w521
      tunnel: w522 -> [w551 w554]
      frame No Error {
        n284 = call "UWB_data_extractor.vi"("Data"=w553) -> ("Z value (mm)"=w546:i32, "Y value (mm)"=w542:i32, "X value (mm)"=w544:i32)  [unwired: 7 in, 1 out]
        n285 = To Double Precision Float(number=w544) -> (double precision float=w543:dbl)
        n286 = Divide(x=w543, y=1000.0) -> (x/y=→"X_UWB":dbl)
        n287 = To Double Precision Float(number=w546) -> (double precision float=w547:dbl)
        n288 = To Double Precision Float(number=w542) -> (double precision float=w541:dbl)
        n289 = Divide(x=w547, y=1000.0) -> (x/y=→"Z_UWB":dbl)
        n290 = Divide(x=w541, y=1000.0) -> (x/y=→"Y_UWB":dbl)
      }
      frame Error {
        n291 = call <vilib>:"Clear Errors.vi"("error in (no error)"=w557, "specific error code to clear (0: all)"=-50400) -> ("error out"=w556:errorcluster)  [unwired: 4 in, 1 out]
      }
    }
    n292 = shared-variable ".\\Shared resources RT.lvlib\\Stop!"() -> (w533:bool)  [unwired: 1 in, 1 out]
    n293 = Or(x=w525, y=w533) -> (x .or. y?=w532:bool)
  }
  n294 = shared-variable ".\\Shared resources RT.lvlib\\Stop!"(w34) -> ()  [unwired: 1 in, 1 out]
  n295 = shared-variable ".\\Shared resources RT.lvlib\\Stop!"(w45) -> ()  [unwired: 1 in, 1 out]
  n296 = shared-variable ".\\Shared resources RT.lvlib\\Stop!"(w19) -> ()  [unwired: 1 in, 1 out]
  n297 = shared-variable ".\\Shared resources RT.lvlib\\Stop!"(w4) -> ()  [unwired: 1 in, 1 out]
  n298 = shared-variable ".\\Shared resources RT.lvlib\\Stop!"(w18) -> ()  [unwired: 1 in, 1 out]
  n299 = Merge Errors(w1, w3) -> (w2:errorcluster)
  n300 = shared-variable ".\\Shared resources RT.lvlib\\Stop!"(w46) -> ()  [unwired: 1 in, 1 out]
  n301 = shared-variable ".\\Shared resources RT.lvlib\\Stop!"(w47) -> ()  [unwired: 1 in, 1 out]
  n302 = Merge Errors(w2, w44, w43) -> (w42:errorcluster)
  n303 = Merge Errors(w42, w53, w52, w51) -> (w50:errorcluster)
  n304 = call "Close Down.vi"("error in (no error)"=w50, "FPGA Interface"=w49) -> ()  [unwired: 9 in, 1 out]
